vi "PH_Timing.PC link GDs.vi"(0 "i ref in":refnum<vi>, 2 "Service Name":string="N/A", 3 "no link":bool, 4 "Status":T1 items=["no info", "off/false/out", "on/true/in", "Failure", "Alarm", "Status 1", "Status 2", "Status 3"], 5 "error in":errorcluster) -> (14 "i ref out":refnum<vi>, 19 "error out":errorcluster)   [LabVIEW 2014, in "PH_Timing.lvlib"]
doc: "This VI writes the incoming information to own attributes and sets GUI elements."
uses:
  PH_Timing.lvlib
  PH_StatusHandler/PH_StatusHandler.Status.ctl
  PH_SRDG645/PH_SRDG645.lvlib
  CSDigitalIO/SRDG535/SRDG535.lvlib
  CSDigitalIO/BNC555/BNC555.lvlib
  PH_StatusHandler/PH_StatusHandler.lvlib
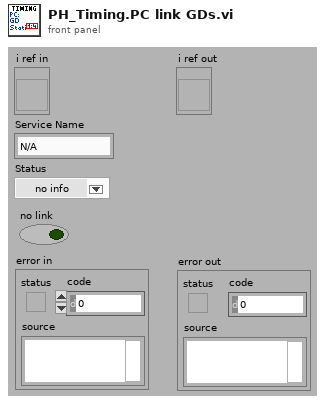
[diagram p1: front panel]
types:
  T1 = typedef "PH_StatusHandler.lvlib/PH_StatusHandler.Status.ctl" = i16
  T2 = typedef "PH_Timing.lvlib/PH_Timing.i attribute.ctl" = cluster{"Sequencer":cluster{"linked?":bool, "Proc State":string, "Ref State":refnum<vi>}, "Gate Generator":cluster{"GD":cluster{"Device Status":T1, "linked?":bool}, "Settings":T3, "GUI Ref":refnum<vi>}, "Interlock Bypass":cluster{"Instancename":string, "Switch linked?":bool, "Device Status":T1, "Ref Status":refnum<vi>}, "Roughtuner":cluster{"Settings":T4, "GUI Ref":refnum<vi>, "GD":cluster{"Device Status":T1, "linked?":bool}}, "0,5Hz Gater":cluster{"Settings":T5, "GUI Ref":refnum<vi>, "GD":cluster{"Device Status":T1, "linked?":bool}}, "Slow Trigger":cluster{"Settings":T6, "GUI Ref":refnum<vi>, "Service ID Delay":i32, "Service ID Ext Trig":i32, "Wanted Settings":T6}, "Timing Mode":cluster{"Mode":T7, "GUI Ref":refnum<vi>, "Service ID T2":i32, "Service ID Mode":i32, "Wanted Mode":T7}, "ns Generator":cluster{"Settings":T8, "ns Generator Settings":refnum<vi>, "GD":cluster{"Device Status":T1, "linked?":bool}}, "Phase FEs":cluster{"Settings":T11, "GUI Ref":refnum<vi>, "Service ID Phase":i32, "Wanted Settings":T11}, "GD GUI Refs":refnum<vi>[], "Heads":T12[], "GUI Ref Delete":refnum<vi>}
  T3 = typedef "PH_Timing.lvlib/PH_Timing.GateGen.ctl" = cluster{"Instance":string, "Channel Gate":i32, "Channel T2":i32, "Width Gate":dbl, "Width T2":dbl, "Delay Gate":dbl, "Delay T2":dbl, "Gate activ":bool, "T2 activ":bool, "System Mode":enum16{"Normal", "Single", "Burst", "Duty Cycle"}}
  T4 = typedef "PH_Timing.lvlib/PH_Timing.Roughtuner.ctl" = cluster{"Instance":string, "Phase PHELIX / UNILAC":cluster{"Channel":u16, "relative to":u16, "Delay [ms]":dbl}, "Pulse Length":cluster{"Channel":u16, "relative to":u16, "Delay [ms]":dbl}, "Trigger":cluster{"externally?":bool, "Rate [Hz]":dbl}}
  T5 = typedef "PH_Timing.lvlib/PH_Timing.0.5HzGater.ctl" = cluster{"Instance":string, "Channel ns FE Delay":i32, "Channel 0.5Hz":i32, "Width ns FE Delay":dbl, "Width 0.5Hz":dbl, "Delay ns FE Delay":dbl, "Delay 0.5Hz":dbl, "ns FE Delay active":bool, "0.5Hz activ":bool, "ns FE Delay inverted":bool, "0.5Hz inverted":bool}
  T6 = typedef "PH_Timing.lvlib/PH_Timing.Slow Trigger Settings.ctl" = cluster{"Delay":dbl, "externally triggered?":bool}
  T7 = typedef "PH_Timing.lvlib/PH_Timing.Timing Mode.ctl" = cluster{"T2":i16, "Modeselector":enum32{"10 Hz", "0.5 Hz", "Shot"}}
  T8 = typedef "PH_Timing.lvlib/PH_Timing.ns Generator.ctl" = cluster{"Instance":string, "Phase fs / ns FE":cluster{"Channel":T9, "Settings":T10}}
  T9 = typedef "Stanford Research DG645 - Driver.lvlib/Channel.ctl" = i32
  T10 = typedef "PH_SRDG645.lvlib/PH_SRDG645.Channel Settings.ctl" = cluster{"Delay [s]":dbl, "relative to":i32}
  T11 = typedef "PH_Timing.lvlib/PH_Timing.Phase FEs.ctl" = cluster{"Phase":dbl}
  T12 = typedef "PH_Timing.lvlib/PH_Timing.PU Data.ctl" = cluster{"linked?":bool, "Data":T13, "GD":cluster{"Device Status":T1, "linked?":bool}, "GUI Ref":refnum<vi>, "PU":T14}
  T13 = typedef "PH_Timing.lvlib/PH_Timing.PU Info.ctl" = cluster{"Act CH?":bool, "GD":string, "CH":i32, "Delay":dbl, "active":bool, "in Use?":bool}
  T14 = typedef "PH_PP_Common.lvlib/PH_PP_Common.PUs.ctl" = enum16{"no Info", "PA-19mm-1", "PA-19mm-2", "PA-45mm-PILC", "PA-45mm-MAIN", "MA-PU-1", "MA-PU-2", "MA-PU-3", "MA-PU-4", "MA-PU-5", "MA-PU-6", "MA-FR", "MA-PILC", "PA-45mm-DP"}
  T15 = enum16{"Normal", "Single", "Burst", "Duty Cycle"}
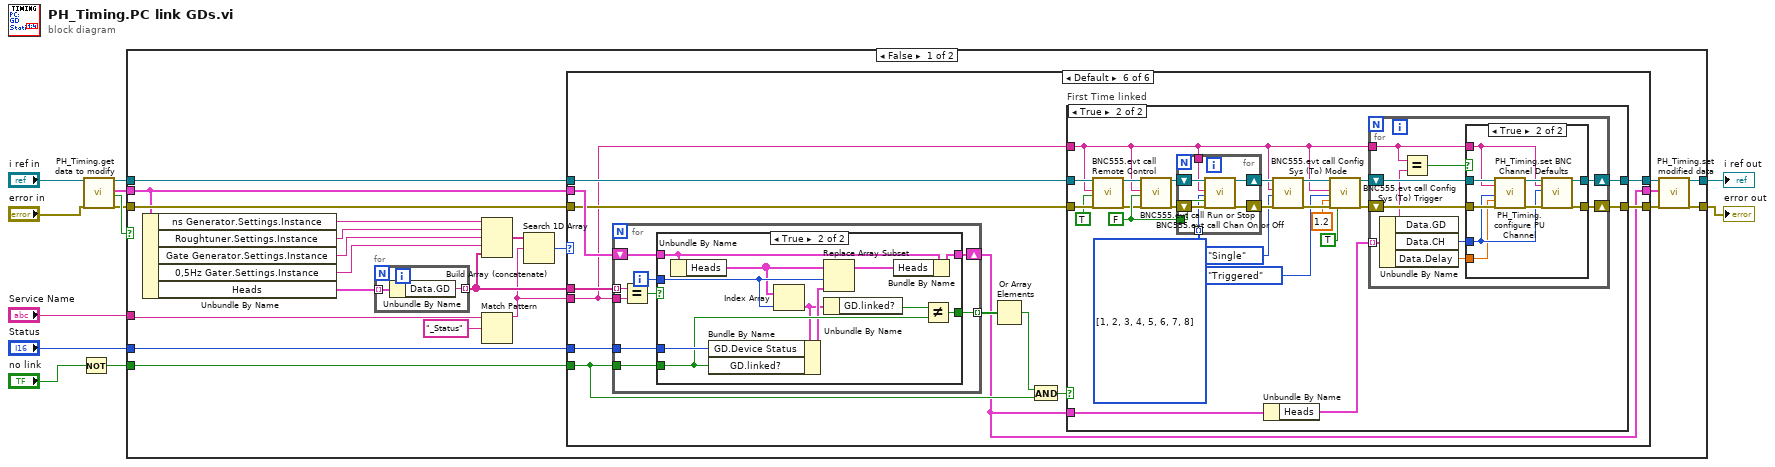
[diagram p0: block diagram]
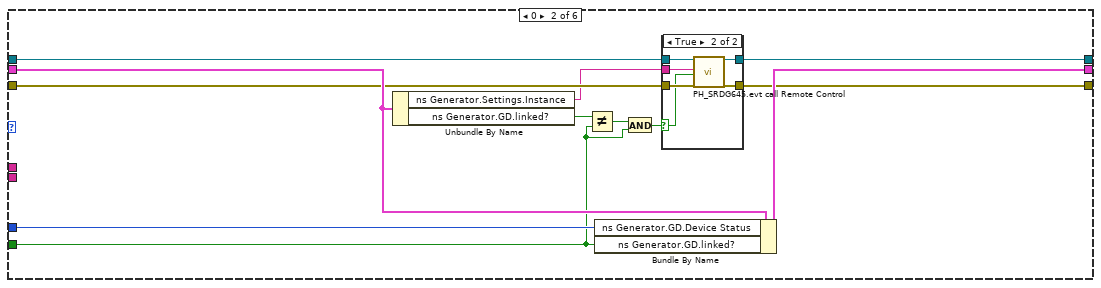
[diagram p3: hidden frame]
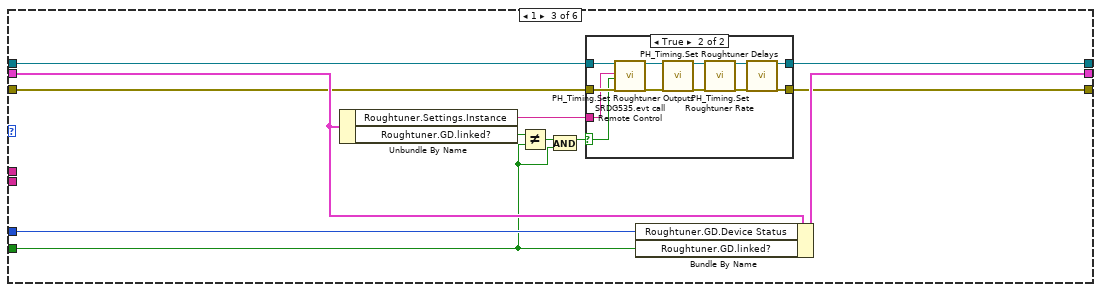
[diagram p5: hidden frame]
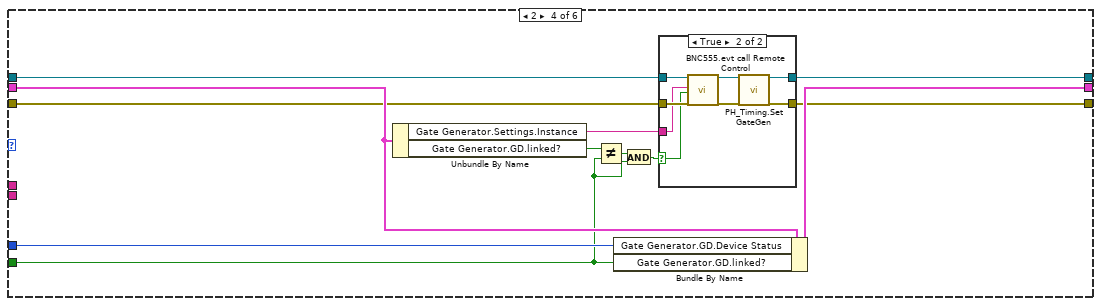
[diagram p7: hidden frame]
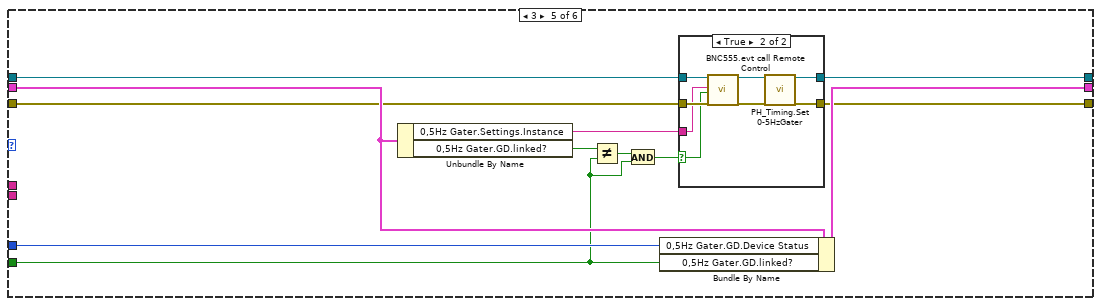
[diagram p9: hidden frame]
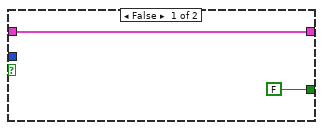
[diagram p13: hidden frame]
diagram:
  n1 = Not(x="no link") -> (.not. x?=w1:bool)
  n2 = call "PH_Timing.get data to modify.vi"("i ref in"="i ref in", "error in (no error)"="error in") -> ("i ref out"=w5:refnum<vi>, "i attribute"=w10:T2, "timed out"=w11:bool, "error out"=w8:errorcluster)  [unwired: 14 in]
  n3 = case shown="False" w11 {
    tunnel: w5 -> [w20 w219]
    tunnel: [w33 w219] -> w6
    tunnel: w8 -> [w29 w218]
    tunnel: [w32 w218] -> w9
    tunnel: w10 -> [w23 _]
    tunnel: w1 -> [w27 _]
    tunnel: "Service Name" -> [w31 _]
    tunnel: "Status" -> [w24 _]
    frame False {
      n4 = Unbundle By Name(w23) -> ("ns Generator.Settings.Instance"=w21:string, "Roughtuner.Settings.Instance"=w18:string, "Gate Generator.Settings.Instance"=w17:string, "0,5Hz Gater.Settings.Instance"=w16:string, "Heads"=w13:T12[])
      n5 = for {
        tunnel: w13 -> [w35] mode=indexing
        tunnel: [w34] -> w15 mode=indexing
        n6 = Unbundle By Name(w35) -> ("Data.GD"=w34:string)
      }
      n7 = Build Array (concatenate)(w21, w18, w17, w16, w15) -> (w22:string[])
      n8 = Match Pattern(string=w31, regular expression="_Status") -> (before substring=w14:string)  [unwired: 1 in, 3 out]
      n9 = Search 1D Array(1D array=w22, element=w14) -> (index of element=w25:i32)  [unwired: 1 in]
      n10 = case shown="Default" w25 {
        tunnel: w29 -> [w38 w43 w62 w88 w111 w136]
        tunnel: [w38 w48 w68 w94 w116 w134] -> w28
        tunnel: w27 -> [_ w39 w59 w85 w107 w132]
        tunnel: w24 -> [_ w49 w69 w95 w117 w139]
        tunnel: w23 -> [w37 w47 w67 w93 w115 w140]
        tunnel: [w37 w50 w70 w96 w118 w131] -> w26
        tunnel: w20 -> [w36 w46 w66 w92 w114 w137]
        tunnel: [w36 w45 w65 w91 w113 w135] -> w19
        tunnel: w15 -> [_ _ _ _ _ w141]
        tunnel: w14 -> [_ _ _ _ _ w133]
        frame -1 {
        }
        frame 0 {
          n11 = Unbundle By Name(w47) -> ("ns Generator.Settings.Instance"=w42:string, "ns Generator.GD.linked?"=w44:bool)
          n12 = Not Equal?(x=w44, y=w39) -> (x != y?=w40:bool)
          n13 = Bundle By Name(cluster=w47, "ns Generator.GD.Device Status"=w49, "ns Generator.GD.linked?"=w39) -> (w50:T2)
          n14 = And(x=w40, y=w39) -> (x .and. y?=w41:bool)
          n15 = case shown="True" w41 {
            selector: w41 -> [_ w53]
            tunnel: w43 -> [w51 w58]
            tunnel: [w51 w57] -> w48
            tunnel: w42 -> [_ w56]
            tunnel: w46 -> [w52 w55]
            tunnel: [w52 w54] -> w45
            frame False {
            }
            frame True {
              n16 = call "PH_SRDG645.evt call Remote Control.vi"("i ref in"=w55, "Generator Instance"=w56, "Remote controlled?"=w53, "error in (no error)"=w58) -> ("i ref out"=w54:refnum<vi>, "error out"=w57:errorcluster)  [unwired: 14 in]
            }
          }
        }
        frame 1 {
          n17 = Unbundle By Name(w67) -> ("Roughtuner.Settings.Instance"=w61:string, "Roughtuner.GD.linked?"=w64:bool)
          n18 = Not Equal?(x=w64, y=w59) -> (x != y?=w63:bool)
          n19 = And(x=w63, y=w59) -> (x .and. y?=w60:bool)
          n20 = case shown="True" w60 {
            selector: w60 -> [_ w77]
            tunnel: w62 -> [w71 w84]
            tunnel: [w71 w78] -> w68
            tunnel: w61 -> [_ w83]
            tunnel: w66 -> [w72 w82]
            tunnel: [w72 w80] -> w65
            frame False {
            }
            frame True {
              n21 = call "SRDG535.evt call Remote Control.vi"("i ref in"=w82, "Generator Instance"=w83, "Remote controlled?"=w77, "error in (no error)"=w84) -> ("i ref out"=w81:refnum<vi>, "error out"=w79:errorcluster)  [unwired: 14 in]
              n22 = call "PH_Timing.Set Roughtuner Outputs.vi"("i ref in"=w81, "error in (no error)"=w79) -> ("i ref out"=w75:refnum<vi>, "error out"=w74:errorcluster)  [unwired: 16 in]
              n23 = call "PH_Timing.Set Roughtuner Rate.vi"("i ref in"=w75, "error in (no error)"=w74) -> ("i ref out"=w76:refnum<vi>, "error out"=w73:errorcluster)  [unwired: 16 in]
              n24 = call "PH_Timing.Set Roughtuner Delays.vi"("i ref in"=w76, "error in"=w73) -> ("i ref out"=w80:refnum<vi>, "error out"=w78:errorcluster)  [unwired: 16 in]
            }
          }
          n25 = Bundle By Name(cluster=w67, "Roughtuner.GD.Device Status"=w69, "Roughtuner.GD.linked?"=w59) -> (w70:T2)
        }
        frame 2 {
          n26 = Unbundle By Name(w93) -> ("Gate Generator.Settings.Instance"=w87:string, "Gate Generator.GD.linked?"=w90:bool)
          n27 = Not Equal?(x=w90, y=w85) -> (x != y?=w89:bool)
          n28 = Bundle By Name(cluster=w93, "Gate Generator.GD.Device Status"=w95, "Gate Generator.GD.linked?"=w85) -> (w96:T2)
          n29 = And(x=w89, y=w85) -> (x .and. y?=w86:bool)
          n30 = case shown="True" w86 {
            selector: w86 -> [_ w99]
            tunnel: w88 -> [w97 w105]
            tunnel: [w97 w100] -> w94
            tunnel: w87 -> [_ w104]
            tunnel: w92 -> [w98 w106]
            tunnel: [w98 w102] -> w91
            frame False {
            }
            frame True {
              n31 = call "BNC555.evt call Remote Control.vi"("i ref in"=w106, "Generator Instance"=w104, "Remote controlled?"=w99, "error in (no error)"=w105) -> ("i ref out"=w103:refnum<vi>, "error out"=w101:errorcluster)  [unwired: 14 in]
              n32 = call "PH_Timing.Set GateGen.vi"("i ref in"=w103, "error in (no error)"=w101) -> ("i ref out"=w102:refnum<vi>, "error out"=w100:errorcluster)  [unwired: 16 in]
            }
          }
        }
        frame 3 {
          n33 = Unbundle By Name(w115) -> ("0,5Hz Gater.Settings.Instance"=w110:string, "0,5Hz Gater.GD.linked?"=w112:bool)
          n34 = Not Equal?(x=w112, y=w107) -> (x != y?=w108:bool)
          n35 = And(x=w108, y=w107) -> (x .and. y?=w109:bool)
          n36 = Bundle By Name(cluster=w115, "0,5Hz Gater.GD.Device Status"=w117, "0,5Hz Gater.GD.linked?"=w107) -> (w118:T2)
          n37 = case shown="True" w109 {
            selector: w109 -> [_ w121]
            tunnel: w111 -> [w119 w127]
            tunnel: [w119 w122] -> w116
            tunnel: w110 -> [_ w126]
            tunnel: w114 -> [w120 w128]
            tunnel: [w120 w124] -> w113
            frame False {
            }
            frame True {
              n38 = call "BNC555.evt call Remote Control.vi"("i ref in"=w128, "Generator Instance"=w126, "Remote controlled?"=w121, "error in (no error)"=w127) -> ("i ref out"=w125:refnum<vi>, "error out"=w123:errorcluster)  [unwired: 14 in]
              n39 = call "PH_Timing.Set 0-5HzGater.vi"("i ref in"=w125, "error in (no error)"=w123) -> ("i ref out"=w124:refnum<vi>, "error out"=w122:errorcluster)  [unwired: 16 in]
            }
          }
        }
        frame Default {
          n40 = for {
            tunnel: w141 -> [w204] mode=indexing
            tunnel: w133 -> [w203]
            shift-right: [w199] -> w131
            shift-left: w140 -> [w200]
            tunnel: w132 -> [w198]
            tunnel: w139 -> [w197]
            tunnel: [w196] -> w138 mode=indexing
            i -> [w202]
            n41 = Equal?(x=w204, y=w203) -> (x = y?=w201:bool)
            n42 = case shown="True" w201 {
              tunnel: w202 -> [_ w215]
              tunnel: w200 -> [w206 w216]
              tunnel: [w206 w217] -> w199
              tunnel: w198 -> [_ w212]
              tunnel: w197 -> [_ w214]
              tunnel: [FALSE w211] -> w196
              frame False {
              }
              frame True {
                n43 = Unbundle By Name(w216) -> ("Heads"=w208:T12[])
                n44 = Index Array(array=w208, index=w215) -> (element=w209:T12)
                n45 = Bundle By Name(cluster=w209, "GD.Device Status"=w214, "GD.linked?"=w212) -> (w210:T12)
                n46 = Replace Array Subset(array=w208, new element=w210, index=w215) -> (w207:T12[])
                n47 = Unbundle By Name(w209) -> ("GD.linked?"=w213:bool)
                n48 = Bundle By Name(cluster=w216, "Heads"=w207) -> (w217:T2)
                n49 = Not Equal?(x=w213, y=w212) -> (x != y?=w211:bool)
              }
            }
          }
          n50 = Or Array Elements(Boolean array=w138) -> (logical OR=w129:bool)
          n51 = And(x=w129, y=w132) -> (x .and. y?=w130:bool)
          n52 = case "First Time linked" shown="True" w130 {
            tunnel: w137 -> [w143 w150]
            tunnel: w136 -> [w142 w148]
            tunnel: [w143 w154] -> w135
            tunnel: [w142 w153] -> w134
            tunnel: w133 -> [_ w146]
            tunnel: w131 -> [_ w151]
            frame False {
            }
            frame True {
              w152 = i32[] [1, 2, 3, 4, 5, 6, 7, 8] items=["System (To)", "Channel A", "Channel B", "Channel C", "Channel D", "Channel E", "Channel F", "Channel G", "Channel H"]
              w165 = FALSE
              n53 = call "BNC555.evt call Remote Control.vi"("i ref in"=w150, "Generator Instance"=w146, "Remote controlled?"=TRUE, "error in (no error)"=w148) -> ("i ref out"=w149:refnum<vi>, "error out"=w147:errorcluster)  [unwired: 14 in]
              n54 = call "BNC555.evt call Run or Stop.vi"("i ref in"=w149, "Generator Instance"=w146, "Start\\Stop"=w165, "error in (no error)"=w147) -> ("i ref out"=w163:refnum<vi>, "error out"=w164:errorcluster)  [unwired: 14 in]
              n55 = for {
                tunnel: w165 -> [w171]
                shift-right: [w169] -> w166
                shift-left: w163 -> [w173]
                shift-right: [w168] -> w167
                shift-left: w164 -> [w174]
                tunnel: w146 -> [w172]
                tunnel: w152 -> [w170] mode=indexing
                n56 = call "BNC555.evt call Chan On or Off.vi"("i ref in"=w173, "Generator Instance"=w172, "Channel"=w170, "State"=w171, "error in (no error)"=w174) -> ("i ref out"=w169:refnum<vi>, "error out"=w168:errorcluster)  [unwired: 13 in]
              }
              n57 = Unbundle By Name(w151) -> ("Heads"=w144:T12[])
              n58 = call "BNC555.evt call Config Sys (To) Mode.vi"("i ref in"=w166, "Generator Instance"=w146, "Mode"=T15."Single", "error in (no error)"=w167) -> ("i ref out"=w161:refnum<vi>, "error out"=w160:errorcluster)  [unwired: 14 in]
              n59 = call "BNC555.evt call Config Sys (To) Trigger.vi"("i ref in"=w161, "Generator Instance"=w146, "Mode"=enum16{"Disabled", "Triggered", "Gated"}."Triggered", "Trigger Level (2.5V)"=1.2 ("Trigger Level [V] (0.5)"), "error in (no error)"=w160, "Trigger Edge (T:Rising)"=TRUE) -> ("i ref out"=w155:refnum<vi>, "error out"=w156:errorcluster)  [unwired: 12 in]
              n60 = for {
                tunnel: w146 -> [w179]
                shift-right: [w181] -> w154
                shift-left: w155 -> [w184]
                shift-right: [w182] -> w153
                shift-left: w156 -> [w183]
                tunnel: w144 -> [w180] mode=indexing
                n61 = Unbundle By Name(w180) -> ("Data.GD"=w178:string, "Data.CH"=w176:i32, "Data.Delay"=w175:dbl)
                n62 = Equal?(x=w179, y=w178) -> (x = y?=w177:bool)
                n63 = case shown="True" w177 {
                  tunnel: w184 -> [w186 w195]
                  tunnel: w183 -> [w185 w194]
                  tunnel: [w185 w192] -> w182
                  tunnel: [w186 w190] -> w181
                  tunnel: w179 -> [_ w189]
                  tunnel: w176 -> [_ w188]
                  tunnel: w175 -> [_ w187]
                  frame False {
                  }
                  frame True {
                    n64 = call "PH_Timing.configure PU Channel.vi"("i ref in"=w195, "GateGen Instance"=w189, "Channel"=w188, "Delay"=w187, "error in"=w194) -> ("i ref out"=w191:refnum<vi>, "error out"=w193:errorcluster)  [unwired: 13 in]
                    n65 = call "PH_Timing.set BNC Channel Defaults.vi"("i ref in"=w191, "Instancename"=w189, "Channel"=w188, "error in (no error)"=w193) -> ("i ref out"=w190:refnum<vi>, "error out"=w192:errorcluster)  [unwired: 14 in]
                  }
                }
              }
            }
          }
        }
      }
      n66 = call "PH_Timing.set modified data.vi"("i ref in"=w19, "i attribute"=w26, "error in (no error)"=w28) -> ("i ref out"=w33:refnum<vi>, "error out"=w32:errorcluster)  [unwired: 15 in]
    }
    frame True {
    }
  }
  "error out" <- w9
  "i ref out" <- w6
